vi "Turn On-Off 5V.vi"(8 "error in (no error)":errorcluster, 10 "Value":bool=TRUE, 11 "NI-DAQ in":refnum<class "NI-DAQ.lvclass">) -> (0 "error out":errorcluster, 3 "NI-DAQ out":refnum<class "NI-DAQ.lvclass">)   [LabVIEW 2019, in "NI-DAQ.lvclass"]
uses:
  NI-DAQ.lvclass
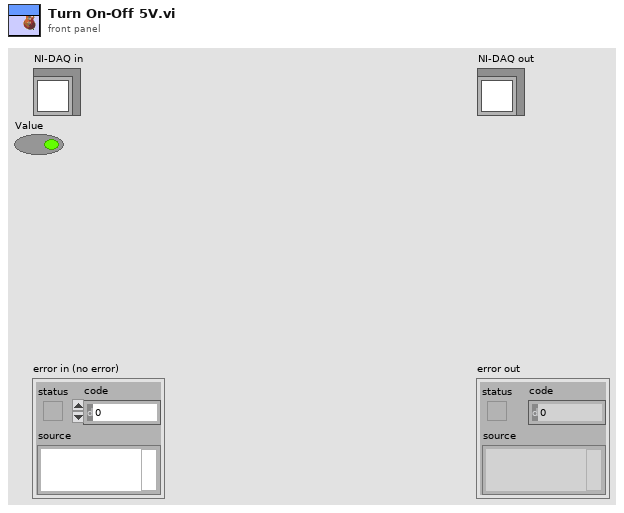
[diagram p1: front panel]
types:
  T1 = typedef "I-O.lvclass/Pin Map.ctl" = cluster{"Region Valves":i32[], "Extra Valves":dbl[][][], "Tool Primary Valve":i32, "Tool Secondary Valve":i32, "Region Sensors":i32[], "Extra Sensors":dbl[][][], "Tool Primary Sensor":dbl, "Tool Secondary Sensor":dbl, "Compression Sensor":dbl, "5V":i32, "Dispener":dbl}
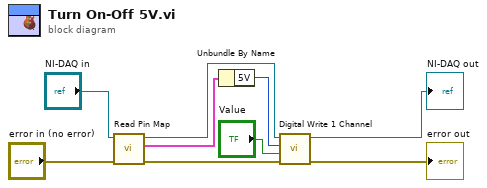
[diagram p0: block diagram]
diagram:
  n1 = call-dynamic "Read Pin Map.vi"("error in (no error)"="error in (no error)", "NI-DAQ in"="NI-DAQ in") -> ("error out"=w5:errorcluster, "Pin Map"=w3:T1, "NI-DAQ out"=w7:refnum<class "NI-DAQ.lvclass">)  [unwired: 7 in]
  n2 = Unbundle By Name(w3) -> ("5V"=w2:i32)
  n3 = call-dynamic "Digital Write 1 Channel.vi"("error constant"=w5, "Value"="Value", "Channel"=w2, "NI-DAQ.lvclass"=w7) -> ("error IO"=→"error out":errorcluster, "NI-DAQ.lvclass 2"=→"NI-DAQ out":refnum<class "NI-DAQ.lvclass">)  [unwired: 6 in]
